vi "generate pulse train.vi"() -> ()   [LabVIEW 2019]
uses:
  <vilib>/DAQmx/create/channels.llb/DAQmx Create Channel (CO-Pulse Generation-Frequency).vi
  <vilib>/DAQmx/configure/timing.llb/DAQmx Timing (Implicit).vi
  <resource>/objmgr/daqmx.rc
panel:
  out "Error Out":errorcluster
  in  "Stop Button":bool
  in  "DAQmx Physical Channel":tag="PXI1Slot7/ctr1"
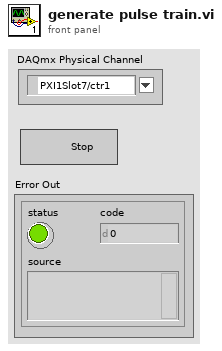
[diagram p1: front panel]
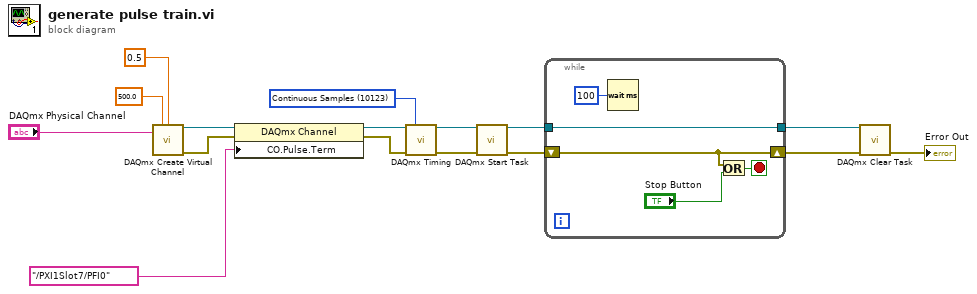
[diagram p0: block diagram]
diagram:
  w1 = 10123 items=["Finite Samples"=10178, "Continuous Samples"=10123, "Hardware Timed Single Point"=12522] ("sample mode")
  n1 = call-poly <vilib>:"DAQmx Create Virtual Channel.vi"("frequency"=500.0, "duty cycle"=0.5, "counter"="DAQmx Physical Channel") -> ("task out"=w8:refnum<k21>, "error out"=w7:errorcluster)  [unwired: 11 in]
  n2 = property class="DAQmx Channel"(reference=w8, error in=w7, "CO.Pulse.Term"=tag "/PXI1Slot7/PFI0") -> (reference out=w5:refnum<k21>, error out=w4:errorcluster)
  n3 = call-poly <vilib>:"DAQmx Timing.vi"("task/channels in"=w5, "sample mode"=w1, "error in"=w4) -> ("task out"=w2:refnum<k21>, "error out"=w3:errorcluster)  [unwired: 11 in]
  n4 = call <vilib>:"DAQmx Start Task.vi"("task/channels in"=w2, "error in"=w3) -> ("task out"=w12:refnum<k21>, "error out"=w13:errorcluster)  [unwired: 12 in]
  n5 = while {
    shift-right: [w21] -> w11
    shift-left: w13 -> [w21]
    tunnel: w12 -> [w18]
    tunnel: [w18] -> w10
    stop <- w19 stop-if-true
    n6 = Wait (ms)(milliseconds to wait=u32 100) -> ()  [unwired: 1 out]
    n7 = Or(x=w21, y="Stop Button") -> (x .or. y?=w19:bool)
  }
  n8 = call <vilib>:"DAQmx Clear Task.vi"("task in"=w10, "error in"=w11) -> ("error out"=→"Error Out":errorcluster)  [unwired: 13 in]
